vi "HelloWorld.vi"   [LabVIEW 2024]
uses:
  Init/Init.lvlib
  Video/Video.lvlib
  Render/Render.lvlib
  Render/PixelFormat--enum.ctl
  Render/TextureAccess-enum.ctl
  Video/WindowFlags--ring.ctl
types:
  T1 = typedef "SDL3.lvlib/Render.lvlib/TextureAccess-enum.ctl" = enum32{"SDL_TEXTUREACCESS_STATIC", "SDL_TEXTUREACCESS_STREAMING", "SDL_TEXTUREACCESS_TARGET"}
  T2 = typedef "SDL3.lvlib/Render.lvlib/PixelFormat--enum.ctl" = enum32{"SDL_PIXELFORMAT_UNKNOWN", "SDL_PIXELFORMAT_INDEX1LSB", "SDL_PIXELFORMAT_INDEX1MSB", "SDL_PIXELFORMAT_INDEX2LSB", "SDL_PIXELFORMAT_INDEX2MSB", "SDL_PIXELFORMAT_INDEX4LSB", "SDL_PIXELFORMAT_INDEX4MSB", "SDL_PIXELFORMAT_INDEX8", "SDL_PIXELFORMAT_RGB332", "SDL_PIXELFORMAT_XRGB4444", "SDL_PIXELFORMAT_XBGR4444", "SDL_PIXELFORMAT_XRGB1555", "SDL_PIXELFORMAT_XBGR1555", "SDL_PIXELFORMAT_ARGB4444", "SDL_PIXELFORMAT_RGBA4444", "SDL_PIXELFORMAT_ABGR4444", "SDL_PIXELFORMAT_BGRA4444", "SDL_PIXELFORMAT_ARGB1555", "SDL_PIXELFORMAT_RGBA5551", "SDL_PIXELFORMAT_ABGR1555", "SDL_PIXELFORMAT_BGRA5551", "SDL_PIXELFORMAT_RGB565", "SDL_PIXELFORMAT_BGR565", "SDL_PIXELFORMAT_RGB24", "SDL_PIXELFORMAT_BGR24", "SDL_PIXELFORMAT_XRGB8888", "SDL_PIXELFORMAT_RGBX8888", "SDL_PIXELFORMAT_XBGR8888", "SDL_PIXELFORMAT_BGRX8888", "SDL_PIXELFORMAT_ARGB8888", "SDL_PIXELFORMAT_RGBA8888", "SDL_PIXELFORMAT_ABGR8888", "SDL_PIXELFORMAT_BGRA8888", "SDL_PIXELFORMAT_XRGB2101010", "SDL_PIXELFORMAT_XBGR2101010", "SDL_PIXELFORMAT_ARGB2101010", "SDL_PIXELFORMAT_ABGR2101010", "SDL_PIXELFORMAT_RGB48", "SDL_PIXELFORMAT_BGR48", "SDL_PIXELFORMAT_RGBA64", "SDL_PIXELFORMAT_ARGB64", "SDL_PIXELFORMAT_BGRA64", "SDL_PIXELFORMAT_ABGR64", "SDL_PIXELFORMAT_RGB48_FLOAT", "SDL_PIXELFORMAT_BGR48_FLOAT", "SDL_PIXELFORMAT_RGBA64_FLOAT", "SDL_PIXELFORMAT_ARGB64_FLOAT", "SDL_PIXELFORMAT_BGRA64_FLOAT", "SDL_PIXELFORMAT_ABGR64_FLOAT", "SDL_PIXELFORMAT_RGB96_FLOAT", "SDL_PIXELFORMAT_BGR96_FLOAT", "SDL_PIXELFORMAT_RGBA128_FLOAT", "SDL_PIXELFORMAT_ARGB128_FLOAT", "SDL_PIXELFORMAT_BGRA128_FLOAT", "SDL_PIXELFORMAT_ABGR128_FLOAT"}
  T3 = typedef "SDL3.lvlib/Video.lvlib/WindowFlags--ring.ctl" = u64
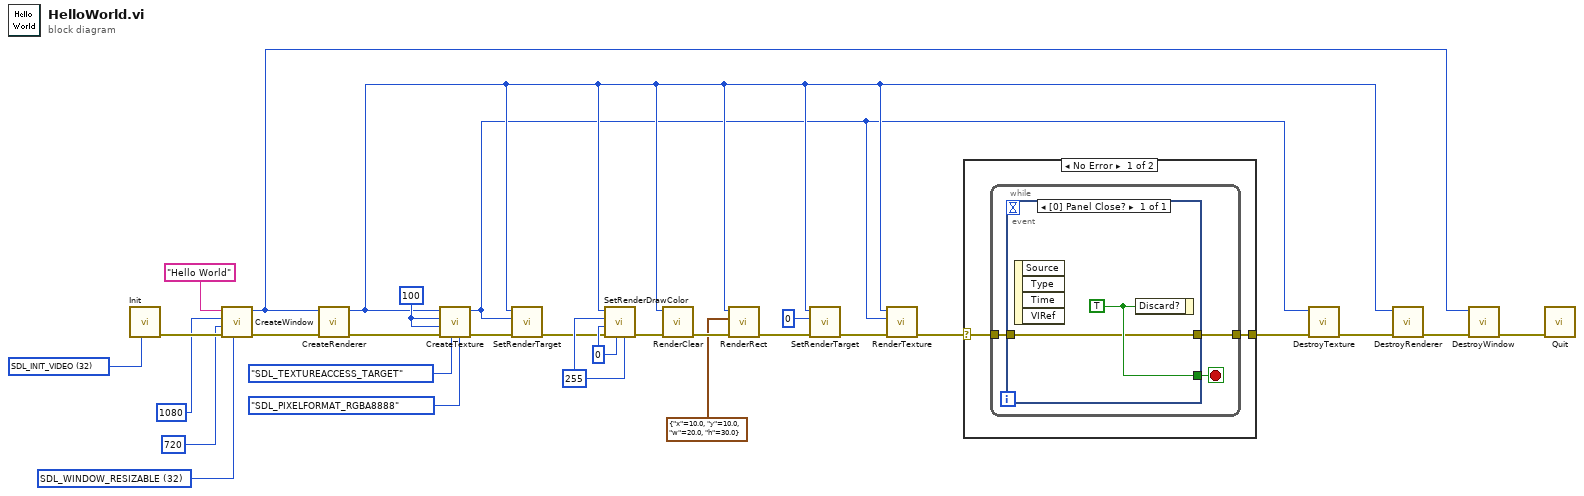
[diagram p0: block diagram]
diagram:
  w12 = u8 0 ("g")
  w11 = u8 255 ("r")
  w17 = 100 ("w")
  w23 = T3 32 items=["0"=0, "SDL_WINDOW_FULLSCREEN"=1, "SDL_WINDOW_OPENGL"=2, "SDL_WINDOW_OCCLUDED"=4, "SDL_WINDOW_HIDDEN"=8, "SDL_WINDOW_BORDERLESS"=16, "SDL_WINDOW_RESIZABLE"=32, "SDL_WINDOW_MINIMIZED"=64, "SDL_WINDOW_MAXIMIZED"=128, "SDL_WINDOW_MOUSE_GRABBED"=256, "SDL_WINDOW_INPUT_FOCUS"=512, "SDL_WINDOW_MOUSE_FOCUS"=1024, "SDL_WINDOW_EXTERNAL"=2048, "SDL_WINDOW_MODAL"=4096, "SDL_WINDOW_HIGH_PIXEL_DENSITY"=8192, "SDL_WINDOW_MOUSE_CAPTURE"=16384, "SDL_WINDOW_MOUSE_RELATIVE_MODE"=32768, "SDL_WINDOW_ALWAYS_ON_TOP"=65536, "SDL_WINDOW_UTILITY"=131072, "SDL_WINDOW_TOOLTIP"=262144, "SDL_WINDOW_POPUP_MENU"=524288, "SDL_WINDOW_KEYBOARD_GRABBED"=1048576, "SDL_WINDOW_VULKAN"=268435456, "SDL_WINDOW_METAL"=536870912, "SDL_WINDOW_TRANSPARENT"=1073741824, "SDL_WINDOW_NOT_FOCUSABLE"=2147483648] ("flags (0)")
  w29 = u32 32 items=["NONE"=0, "SDL_INIT_AUDIO"=16, "SDL_INIT_VIDEO"=32, "SDL_INIT_JOYSTICK"=512, "SDL_INIT_HAPTIC"=4096, "SDL_INIT_GAMEPAD"=8192, "SDL_INIT_EVENTS"=16384, "SDL_INIT_SENSOR"=32768, "SDL_INIT_CAMER"=65536] ("flags")
  n1 = call "Init.vi"("flags (0)"=w29) -> ("error out"=w28:errorcluster)  [unwired: 10 in]
  n2 = call "CreateWindow.vi"("flags (0)"=w23, "No Error"=w28, "h"=720, "w"=1080, "title"="Hello World") -> ("error out"=w22:errorcluster, "window [SDL_Window *]"=w21:i64)  [unwired: 5 in]
  n3 = call "CreateRenderer.vi"("No Error"=w22, "window [SDL_Window *]"=w21) -> ("error out"=w18:errorcluster, "renderer [SDL_Renderer *]"=w2:i64)  [unwired: 8 in]
  n4 = call "CreateTexture.vi"("pixel_format"=PixelFormat--enum."SDL_PIXELFORMAT_RGBA8888", "texture_access"=TextureAccess-enum."SDL_TEXTUREACCESS_TARGET", "No Error"=w18, "h"=w17, "w"=w17, "renderer [SDL_Renderer *]"=w2) -> ("error out"=w13:errorcluster, "texture [SDL_Texture *]"=w1:i64)  [unwired: 4 in]
  n5 = call "SetRenderTarget.vi"("No Error"=w13, "texture [SDL_Texture *]"=w1, "renderer [SDL_Renderer *]"=w2) -> ("error out"=w6:errorcluster)  [unwired: 8 in]
  n6 = call "SetRenderDrawColor.vi"("a"=w11, "b"=w12, "No Error"=w6, "g"=w12, "r"=w11, "renderer [SDL_Renderer *]"=w2) -> ("error out"=w10:errorcluster)  [unwired: 5 in]
  n7 = call "RenderClear.vi"("No Error"=w10, "renderer [SDL_Renderer *]"=w2) -> ("error out"=w9:errorcluster)  [unwired: 9 in]
  n8 = call "RenderRect.vi"("No Error"=w9, "rect"=cluster{"x":sgl, "y":sgl, "w":sgl, "h":sgl} {"x"=10.0, "y"=10.0, "w"=20.0, "h"=30.0}, "renderer [SDL_Renderer *]"=w2) -> ("error out"=w8:errorcluster)  [unwired: 8 in]
  n9 = call "SetRenderTarget.vi"("No Error"=w8, "texture [SDL_Texture *]"=i64 0, "renderer [SDL_Renderer *]"=w2) -> ("error out"=w5:errorcluster)  [unwired: 8 in]
  n10 = call "RenderTexture.vi"("No Error"=w5, "texture [SDL_Texture *]"=w1, "renderer [SDL_Renderer *]"=w2) -> ("error out"=w3:errorcluster)  [unwired: 8 in]
  n11 = case shown="No Error" w3 {
    selector: w3 -> [w31 w37]
    tunnel: [w30 w37] -> w20
    frame No Error {
      n12 = while {
        tunnel: w31 -> [w33]
        tunnel: [w34] -> w30
        stop <- w32 stop-if-true
        n13 = event shown="[0] Panel Close?" {
          selector: _ -> [_]
          dyn-events: _ -> [_]
          timeout: _ -> [_]
          tunnel: [w35] -> w34
          tunnel: w33 -> [w35]
          tunnel: [w36] -> w32
          event Panel Close? {
            w36 = TRUE ("Discard?")
            n14 = event-data() -> ()  [unwired: 1 in, 4 out]
            n15 = event-data("Discard?"=w36) -> ()  [unwired: 1 in, 1 out]
          }
        }
      }
    }
    frame Error {
    }
  }
  n16 = call "DestroyTexture.vi"("No Error"=w20, "texture [SDL_Texture *]"=w1) -> ("error out"=w14:errorcluster)  [unwired: 9 in]
  n17 = call "DestroyRenderer.vi"("No Error"=w14, "renderer [SDL_Renderer *]"=w2) -> ("error out"=w19:errorcluster)  [unwired: 9 in]
  n18 = call "DestroyWindow.vi"("No Error"=w19, "window [SDL_Window*]"=w21) -> ("error out"=w27:errorcluster)  [unwired: 9 in]
  n19 = call "Quit.vi"("No Error"=w27) -> ()  [unwired: 10 in, 1 out]
